vi "SubConfocal_GetFWPos.vi"(7 "Confocal Ref":refnum<vi>, 8 "Error In":errorcluster, 11 "Confocal line (VISA IN)":refnum<visa-resource-name>="COM1") -> (0 "Error out":errorcluster, 3 "VISA OUT":refnum<visa-resource-name>)   [LabVIEW 2015]
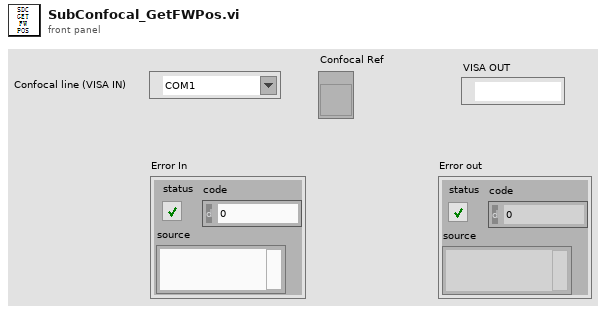
[diagram p1: front panel]
types:
  T1 = cluster{"SDC shutter":bool, "FWPosition":i32, "FW speed":i32, "Disk spinning?":bool, "Disk speed (rpm)":dbl, "Actual speed (rpm)":string}
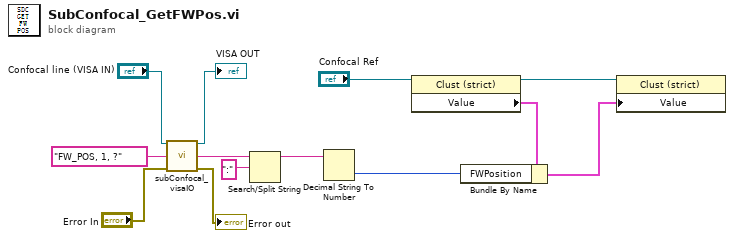
[diagram p0: block diagram]
diagram:
  n1 = call "subConfocal_visaIO.vi"("VISA  IN"="Confocal line (VISA IN)", "Command (to ctlr)"="FW_POS, 1, ?", "error in"="Error In") -> ("VISA OUT"=→"VISA OUT":refnum<visa-resource-name>, "Raw Response"=w13:string, "error out"=→"Error out":errorcluster)  [unwired: 8 in, 2 out]
  n2 = Search/Split String(string=w13, search string/char (-)=":") -> (substring before match=w6:string)  [unwired: 1 in, 2 out]
  n3 = Decimal String To Number(string=w6) -> (number=w1:i32)  [unwired: 2 in, 1 out]
  n4 = property class="Clust (strict)"(reference="Confocal Ref") -> (reference out=w4:refnum<vi>, "Value"=w3:T1)  [unwired: 1 in, 1 out]
  n5 = Bundle By Name(cluster=w3, "FWPosition"=w1) -> (w5:T1)
  n6 = property class="Clust (strict)"(reference=w4, "Value"=w5) -> ()  [unwired: 1 in, 2 out]
